vi "write_init.vi"(8 "error in (no error)":errorcluster, 10 "init":dbl[](array[numeric]), 11 "MDS in":refnum<class "MDS.lvclass">) -> (0 "error out":errorcluster, 3 "MDS out":refnum<class "MDS.lvclass">)   [LabVIEW 2020, in "MDS.lvclass"]
uses:
  MDS.lvclass
  MDS.lvclass/MDS.ctl
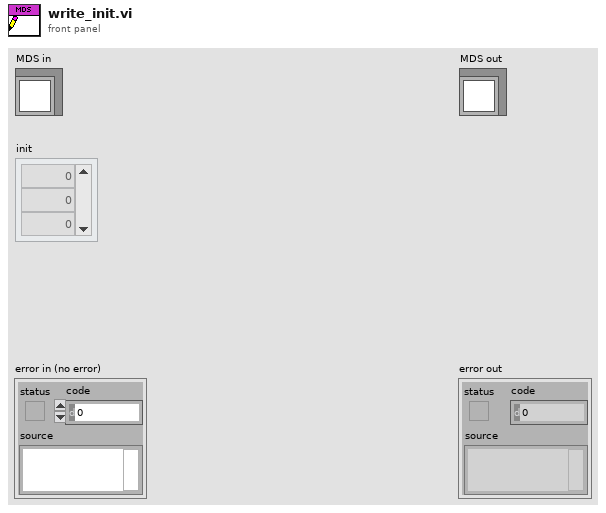
[diagram p1: front panel]
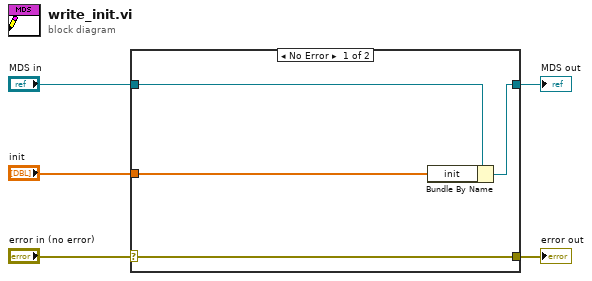
[diagram p0: block diagram]
diagram:
  n1 = case shown="No Error" "error in (no error)" {
    selector: "error in (no error)" -> [w9 w10]
    tunnel: [w9 w10] -> w4
    tunnel: [w7 w11] -> w2
    tunnel: "MDS in" -> [w8 w11]
    tunnel: "init" -> [w6 _]
    frame No Error {
      n2 = Bundle By Name(cluster=w8, "init"=w6) -> (w7:refnum<class "MDS.lvclass">)
    }
    frame Error {
    }
  }
  "error out" <- w4
  "MDS out" <- w2
